vi "Day 2 - part a solution.vi"() -> ()   [LabVIEW 2020]
panel:
  in  "Input":string="A Y\nB X\nB X\nC Y\nB X\nA Z\nB X\nB X\nC Z\nA Z\nC Z\nA X\nA Y\nA Y\nB X\nC Y\nB Z\nA X\nB X\nC Y\nC Y\nA Y\nA Y\nC Y\nB X\nB X\nB X\nA X\nB X\nB X\nC Y\nC Y\nB X\nA Z\nA Z\nB X\nA Z\nC Y\nB X\nB X\nB X\nB X\nB X\nB Z\nA Z\nB X\nA Z\nA X\nB X\nA Z\nB X\nC Y\nA Z\nA Z\nB X\nB X\nB Z\nC Y\nA Y\nB Z\nA Z\nC Z\nB X\nC Y\nC Y\nB Z\nB X\nB X\nB Z\nB X\nB X\nA Y\nA Z\nB Z\nB X\nB Y\nB Z\nB X\nC X\nB Z\nB X\nA Z\nB Z\nB Z\nB X\nA Y\nA Z\nA Y\nB X\nB Z\nB X\nB X\nA Y\nA Y\nB X\nB X\nB X\nC X\nC Y\nB X\nB X\nB Z\nB X\nB X\nB X\nC Y\nB X\nC Y\nA Z\nB X\nB Z\nB X\nC Y\nC Y\nA Z\nA Y\nC Y\nB X\nB X\nB Z\nA Y\nB X\nB X\nB X\nA Y\nB Z\nB X\nA Y\nB Z\nC Y\nA X\nB X\nB X\nA Z\nC Y\nB X\nB Z\nA Y\nA Y\nC Y\nA Y\nC Y\nB X\nB Z\nB X\nC Y\nA Y\nB X\nC Z\nA Z\nC Y\nB X\nB Z\nB X\nB X\nB Z\nB Y\nA Y\nB X\nA Y\nA Z\nA Z\nB X\nC Y\nB Z\nA X\nA Y\nB X\nA Z\nB X\nA Y\nB Y\nB X\nA Y\nB X\nB X\nB X\nB X\nB X\nB X\nB X\nA Z\nB X\nB X\nB Z\nB Z\nB Z\nB Z\nA Y\nB Z\nC Z\nB X\nB X\nB X\nA Z\nB Z\nC Y\nB X\nC Y\nB Z\nB X\nB Z\nB X\nC Z\nA Z\nA Y\nA X\nB X\nB Z\nA Y\nB X\nB X\nB X\nB X\nC Y\nC Y\nA Z\nA Y\nA X\nB X\nB X\nA Y\nB X\nC Y\nA X\nB X\nB X\nB X\nA Z\nC Y\nB Z\nC Y\nA Y\nC Y\nA X\nA Z\nC Z\nA Z\nB X\nB Z\nB X\nB X\nA X\nB X\nB X\nB Z\nA Y\nC Y\nA Z\nC Z\nA Z\nA Z\nA Z\nB Z\nB Z\nB Z\nC Z\nB Y\nC Y\nC Y\nC X\nB X\nC Y\nB X\nB X\nC Y\nB Z\nB X\nC Z\nB X\nA Z\nB Z\nC X\nC Y\nB X\nA Y\nA Z\nB X\nA Z\nA Z\nB X\nB X\nC Z\nB Z\nA Z\nA Z\nC Z\nB X\nA Z\nA X\nB X\nB X\nC Y\nB X\nB Z\nA Z\nB X\nB X\nB X\nB X\nB X\nB X\nB X\nB X\nC Y\nC Y\nB X\nB X\nB X\nC Y\nA X\nB Z\nB X\nB X\nC Z\nB X\nB Z\nB Z\nA Z\nB X\nB Z\nB X\nA Z\nB X\nB X\nB X\nB X\nB X\nC Z\nB X\nB X\nB X\nB Z\nC Y\nC Y\nA Y\nB X\nB Z\nC Y\nB X\nB X\nC Y\nC Y\nB X\nB X\nB X\nB X\nC X\nB Z\nB X\nB Z\nC Y\nA X\nA Z\nB X\nB X\nA Z\nB X\nC Z\nB X\nA Y\nA Z\nB X\nB X\nB X\nB Z\nB X\nA Y\nC Y\nB Z\nB Z\nC Y\nB X\nA Y\nC Y\nB X\nC Z\nB X\nB X\nA Z\nB Z\nB Z\nB X\nA Z\nA Z\nA Y\nB Z\nB X\nB X\nB X\nB X\nB Z\nB X\nB Z\nB X\nA Z\nB X\nB X\nC Z\nC Z\nB X\nC Y\nA Z\nB X\nB Z\nC Z\nC X\nB X\nA Y\nA Y\nB X\nB X\nC Y\nA X\nC Y\nA Y\nA Z\nC Z\nB Z\nA Z\nB X\nB X\nB Z\nC Y\nA Y\nA Y\nB Z\nA Z\nA Z\nB Z\nA Z\nB X\nA Y\nA Y\nC Y\nB X\nB X\nA X\nB X\nC X\nA Y\nA Z\nB X\nB X\nB X\nB X\nB X\nB Z\nB Z\nB Z\nB X\nB X\nA Z\nB X\nC Z\nA Z\nC Y\nB Z\nC Y\nA Y\nC Y\nB X\nB X\nB X\nA Y\nB Z\nB Z\nB X\nB Z\nB X\nB X\nB X\nC Y\nB X\nB Z\nA Z\nB X\nB X\nB X\nC Z\nC Z\nB Z\nB X\nA Z\nA X\nB X\nB X\nB Y\nA Y\nB X\nB X\nC Z\nA Z\nB X\nB Z\nB Z\nA Y\nA Z\nB Z\nB Z\nA Y\nA Y\nA Z\nC Y\nC Y\nB X\nB X\nA Z\nB X\nC Y\nC X\nA Z\nB X\nB X\nB X\nA Y\nC Y\nB Y\nC Y\nC X\nA X\nA Y\nB Z\nB X\nB Z\nA X\nB X\nC Z\nB X\nB X\nA Y\nB Z\nB X\nA Y\nA Y\nB X\nC Y\nB X\nB X\nC Y\nB X\nC Z\nB Z\nB X\nA X\nC Y\nC Y\nB X\nB Z\nB X\nB X\nA Z\nB X\nA Z\nB Z\nB X\nB X\nB Z\nA Y\nC Y\nB Z\nB X\nA Y\nB X\nA X\nC Z\nB X\nB Z\nB Z\nA X\nC Y\nA Z\nB X\nB Z\nA Y\nB X\nC Y\nA Y\nB Z\nC Y\nB X\nB X\nB X\nB X\nB X\nB X\nC Y\nB X\nC Z\nA Y\nC Y\nB X\nC Y\nB Z\nB X\nA X\nB Z\nB X\nC X\nB X\nA Z\nB X\nA Y\nB X\nC Z\nB X\nB Z\nA Y\nB X\nA Z\nA Z\nA Z\nA Y\nA Y\nB X\nA Z\nB X\nB X\nA Y\nA Y\nA Y\nB Z\nC Y\nB Z\nB X\nC Z\nA Y\nC Y\nB X\nB X\nB Z\nB X\nB X\nB X\nC Y\nC Y\nA Y\nB Z\nB Z\nB X\nB X\nB Z\nB X\nA Y\nC Y\nB X\nC X\nB Z\nB X\nB Z\nB Z\nC Y\nB Z\nB X\nC X\nB X\nC Y\nB X\nA Z\nB X\nB X\nB X\nB X\nB X\nC Y\nA Y\nB X\nC Y\nB Z\nB Z\nB X\nC X\nB Z\nC Y\nC X\nC Y\nA Z\nB Z\nC Y\nC X\nB X\nA Y\nC Y\nB X\nC Z\nB Z\nA Y\nC Z\nC X\nB X\nB X\nA Y\nC X\nB X\nB X\nA X\nA Z\nA X\nA Y\nA Y\nC Y\nB X\nC Z\nB X\nC Y\nA Y\nB X\nB X\nB X\nB X\nA Z\nC X\nB X\nB Z\nB X\nB X\nC Y\nB X\nC Z\nB X\nB X\nB X\nB X\nB X\nC Y\nB X\nB X\nA Y\nB X\nC Y\nC Y\nA Y\nB X\nA X\nA Y\nB X\nB Z\nB X\nB Z\nA X\nA Y\nA X\nB X\nC Z\nA Y\nB Z\nA Y\nB Z\nB Z\nB X\nB Z\nB X\nB X\nB X\nB Z\nB X\nB X\nB X\nA Z\nC Z\nC Z\nA X\nA X\nB X\nB X\nA X\nB X\nA X\nA Z\nB Z\nB X\nC Y\nB X\nC Y\nA Y\nC X\nA X\nA Y\nB Z\nB X\nB X\nC Z\nB Y\nA Y\nB Y\nC Y\nA Y\nB X\nB X\nC X\nB Z\nA Y\nB Z\nA Z\nB X\nB X\nA Z\nC Z\nA Y\nB X\nB X\nB Z\nB X\nB X\nB Z\nA X\nA Z\nC Y\nA Y\nA Z\nB X\nC Y\nB Z\nC Y\nB X\nB X\nB Z\nB X\nA Y\nB X\nA Y\nB X\nA Y\nB X\nA Y\nC Y\nA Y\nB Z\nA Y\nB X\nA Z\nC Y\nB X\nB X\nB X\nA X\nB X\nB Z\nA Z\nA Z\nB X\nB Z\nB X\nA Y\nB Z\nB X\nB X\nA Y\nA Y\nC Z\nC Y\nB X\nA X\nA Y\nA X\nC Y\nB X\nC X\nB X\nB X\nA Y\nA Y\nA Y\nB Y\nB X\nB X\nB X\nC Z\nB Z\nC Z\nA X\nB X\nB X\nA Y\nA Z\nB X\nA Y\nB Z\nB Z\nC Y\nB X\nB X\nC X\nB X\nC X\nB X\nB Z\nA X\nB X\nA Z\nA X\nB Z\nA Y\nB X\nB X\nB X\nB X\nB Z\nA Z\nB X\nB Z\nB X\nB Z\nC Y\nB X\nC Y\nB X\nB X\nB X\nA Y\nB X\nA Y\nB X\nB X\nA X\nC Z\nC Y\nA Z\nB X\nA Y\nC Z\nC Y\nC Y\nB Z\nA Y\nB X\nA Y\nB X\nB X\nB Z\nB Z\nB X\nC X\nB Z\nA X\nA Y\nA Y\nB Z\nA Z\nC Y\nB X\nB Z\nA Y\nC Y\nA Y\nA X\nA Z\nB X\nB X\nC Y\nB X\nC Y\nB X\nA X\nB Z\nC X\nB Y\nA Y\nC Y\nB X\nA X\nB X\nB X\nB X\nA Z\nA Y\nB X\nC Z\nB X\nC X\nC Z\nB X\nB X\nC Y\nB X\nB Z\nA Y\nA Y\nB X\nB X\nB Z\nC Y\nB X\nB X\nB X\nA Y\nC Y\nB X\nA Y\nA Z\nC Y\nB X\nA Y\nA Z\nB Z\nA Z\nB X\nC X\nB Z\nA Y\nB Z\nA Y\nC Y\nA X\nA Y\nB X\nC Y\nC Y\nB X\nA X\nB Z\nB X\nB X\nA Z\nA Z\nA Y\nA Y\nB X\nB X\nB X\nA X\nB X\nB X\nB X\nA X\nB Z\nC Z\nA Y\nC Y\nC Y\nC X\nB X\nB Z\nB Z\nB X\nB X\nC Y\nA X\nC Y\nA X\nB X\nB X\nB Z\nB Z\nC Y\nC Y\nA Z\nC Y\nA Z\nB X\nA Z\nA Y\nB Z\nB Z\nB X\nB X\nA Y\nB Z\nB X\nC Z\nA Z\nB Z\nB X\nB Z\nB X\nC Y\nB X\nA Y\nB Z\nC Y\nB Z\nC Z\nB X\nC Z\nB X\nB X\nB X\nC Y\nB X\nB X\nB Z\nA Y\nB X\nB Z\nA Z\nB X\nC Y\nC X\nC Y\nA Z\nB X\nA Z\nB X\nC Z\nA Y\nB Z\nB Z\nA Y\nC Z\nC X\nA Y\nB X\nB Z\nB X\nB X\nB X\nB X\nA X\nB X\nB X\nA Z\nB X\nB X\nA Z\nC Y\nA X\nB Z\nB X\nB X\nA Z\nB X\nA Y\nB Z\nC Y\nB X\nA Y\nC Y\nB Z\nB X\nA Z\nA Z\nB X\nB X\nB Z\nB X\nB X\nA Z\nB X\nB Z\nB Z\nC Y\nA Z\nB X\nA Y\nB X\nB X\nB X\nB Z\nA X\nC Y\nB Z\nB X\nB X\nB X\nB X\nB X\nB Z\nB X\nB Z\nA Z\nB Z\nB X\nC Z\nB Z\nC Z\nA Z\nC X\nA Y\nB Z\nB Z\nB X\nB Z\nB Z\nA Z\nC Z\nA X\nC Y\nC Y\nA Y\nA X\nA Z\nB X\nA Y\nB X\nB X\nC Y\nC Y\nB X\nB Z\nA Y\nB X\nB Z\nB X\nB X\nA Z\nC Y\nB X\nC Y\nA Y\nB Z\nA Z\nA Y\nB X\nA Z\nB Z\nB X\nA Y\nA Y\nA Z\nA X\nB Z\nC Z\nB X\nC Z\nB X\nB Z\nA X\nB X\nB X\nB X\nB X\nC Y\nB X\nA X\nB Z\nA Y\nB X\nA Z\nB X\nB Z\nA Y\nA Y\nA Y\nA Y\nA Z\nC Y\nC Z\nB X\nB Z\nA Y\nB X\nB X\nB X\nA Y\nB Z\nB X\nB Z\nB X\nB X\nB X\nC Y\nC Y\nC X\nB X\nA Y\nA Y\nC Z\nA Y\nA Y\nC X\nA Z\nB X\nB X\nB X\nB X\nC Y\nA Y\nB Z\nA Z\nB X\nC X\nA Z\nB X\nC Y\nB X\nB X\nC Y\nB X\nB X\nB X\nA Y\nB X\nB X\nC Z\nB X\nC Y\nC Y\nB X\nA Z\nB X\nB X\nC Y\nA Y\nB X\nB Z\nB X\nB X\nB X\nC Y\nC Z\nB Z\nC Y\nB X\nB Z\nB X\nB X\nB X\nC Y\nC X\nB X\nA Y\nA Z\nB Z\nA Y\nB X\nB X\nB Y\nC Y\nC X\nB Z\nA Z\nB X\nB X\nA Y\nC Z\nC Y\nB X\nC Y\nA Z\nA Y\nB Z\nB X\nB X\nB X\nB X\nA Z\nA X\nA X\nA X\nC Y\nB Z\nB X\nC Y\nB X\nB X\nA Z\nC Z\nC Z\nB X\nA Y\nB X\nB Z\nB X\nA Y\nA Y\nA Z\nC Y\nA Y\nA Z\nA Y\nA Y\nB X\nA Y\nB X\nA Z\nA Z\nC Y\nB X\nB X\nC Y\nB X\nB X\nB X\nC Y\nA Y\nB X\nA Y\nB Z\nC Y\nB X\nA Y\nB Z\nA Z\nB Z\nA Z\nB X\nC Y\nB X\nB X\nB X\nC Y\nA Y\nB X\nA Y\nC X\nA Z\nB X\nB Y\nB X\nB X\nA Z\nB X\nB X\nB Z\nB X\nC Y\nB X\nB X\nB Z\nB X\nC Y\nB X\nC Y\nB X\nB Z\nA Y\nB X\nB X\nC Z\nB X\nC Y\nA Y\nC Y\nB X\nB Z\nB X\nB X\nB X\nB X\nA Y\nB X\nA Z\nA Y\nA X\nC Y\nB X\nC Y\nB X\nA Z\nC Y\nC Y\nB Z\nB X\nA Y\nB Z\nA Y\nA Y\nB Z\nB Z\nB X\nC Y\nC Y\nB X\nA X\nA Z\nB X\nC Y\nB X\nB X\nB Z\nB X\nB Z\nC Y\nC Z\nC Y\nA Y\nA Z\nB X\nC Y\nA Y\nC X\nB X\nB X\nA Y\nB X\nB X\nB X\nB Z\nB Y\nA X\nA Y\nC Y\nC Y\nA Y\nC Y\nB Z\nB Z\nC Y\nB X\nC Y\nC Z\nA Y\nC X\nA Y\nA Y\nC Y\nC Y\nB X\nA Y\nA X\nB X\nB X\nB Z\nB X\nA Z\nA Y\nA Y\nB X\nB X\nB Z\nB Z\nB X\nB Z\nA Z\nA Y\nA Z\nB X\nC Y\nB Z\nB X\nA Y\nB X\nC X\nB X\nB X\nC Y\nB X\nB X\nB X\nA Y\nA X\nA Y\nB X\nB X\nA Y\nA Y\nA Z\nA Z\nC X\nC Y\nA Z\nC Y\nB Z\nB X\nA Y\nB X\nB Z\nC Z\nA Y\nA Z\nA Y\nB X\nB Z\nB X\nA X\nB Z\nB X\nC Y\nB X\nA Z\nC Z\nA X\nB X\nB X\nA Y\nC Y\nB X\nB X\nB X\nB X\nB X\nA X\nB X\nA Z\nC Z\nB Z\nB X\nC X\nA X\nC Y\nA Y\nA Z\nB X\nA X\nA Z\nA Z\nB X\nB X\nA Z\nC Y\nA Z\nB X\nC Y\nB X\nC Z\nC Y\nC X\nA Z\nC X\nB Z\nB X\nB X\nC Y\nB X\nC Y\nA Z\nA Z\nA Z\nA Y\nA Z\nB X\nB X\nB X\nB Z\nC Y\nC Z\nC Y\nC Y\nC Y\nA Y\nB Z\nA X\nB X\nB X\nB X\nA X\nA Y\nB X\nB Z\nA Z\nA Y\nA Y\nB Z\nB X\nB X\nC Y\nC Y\nC Y\nB X\nC Y\nB X\nB X\nB X\nC Y\nA Y\nA Y\nC Z\nC Y\nB X\nA X\nA Y\nB X\nC Y\nB X\nA Y\nC Y\nA Y\nB X\nB X\nB Z\nA Y\nB Z\nB Z\nB X\nB X\nC X\nC Y\nB X\nB X\nA X\nC Y\nB X\nB Z\nB X\nB X\nA Y\nB X\nB Z\nB Z\nC Y\nB X\nB Z\nB Z\nB Z\nB X\nB X\nA Y\nB X\nB X\nB Z\nC Y\nA Y\nB X\nB Z\nB X\nB X\nA X\nB X\nB X\nB X\nB Z\nB Z\nB Z\nB X\nA Z\nB X\nA Z\nA Y\nB Z\nB X\nA Y\nB X\nB Z\nB X\nA Z\nB X\nB Z\nC Z\nA X\nB X\nB X\nB X\nC Y\nB X\nB X\nA Y\nA Z\nB X\nC Y\nB X\nC Y\nB X\nB Y\nB X\nC Z\nB X\nC Z\nA Y\nB X\nC Z\nB X\nA Y\nC Y\nB X\nB X\nB Z\nC X\nB Z\nB X\nA Z\nB X\nB X\nB X\nB Z\nB X\nA Z\nC Y\nA Y\nB X\nB X\nA Z\nB X\nA Y\nB X\nC Y\nB Z\nB Z\nB X\nB Z\nB X\nB X\nB X\nB X\nB X\nC Y\nA Z\nA Z\nB Z\nA Y\nB Z\nC Y\nA Y\nA Y\nC Y\nA Y\nB Z\nA Y\nA Y\nB X\nB X\nA X\nB X\nC Y\nC Y\nB Z\nB X\nA Z\nB Z\nB X\nA Z\nB Z\nA Y\nA Y\nA Y\nA Y\nA Z\nA Y\nB X\nB Z\nA Y\nB X\nA Z\nB Z\nC X\nB X\nB X\nB Z\nB Z\nB X\nB X\nB X\nB X\nB X\nB X\nB X\nB Z\nB X\nB X\nB X\nB X\nB X\nB Z\nB X\nB X\nB Z\nB Z\nB X\nA Y\nB Z\nB X\nA Z\nA Y\nA Z\nB X\nB X\nA X\nB Y\nA Z\nB X\nC Z\nA Z\nB X\nB Z\nB X\nB X\nB X\nA Y\nC Y\nB X\nB X\nB X\nA Y\nB X\nA Z\nB X\nB X\nB X\nB Z\nB Z\nC X\nC Y\nB X\nB X\nC Y\nB X\nB X\nB X\nA X\nA Z\nA Z\nB Z\nB Z\nB X\nA Y\nB X\nC Y\nB Z\nC Y\nC Z\nA Y\nA Y\nB X\nB X\nA Z\nB X\nB X\nB Z\nB X\nB X\nA Z\nB X\nB X\nB X\nC Y\nB X\nB X\nC Y\nB X\nB X\nB Z\nB X\nB X\nA Y\nC Y\nA X\nC Y\nB X\nB X\nA Z\nA Y\nB X\nA X\nB Z\nA Y\nB X\nB X\nA Y\nB X\nC X\nB X\nB X\nB Z\nB Z\nB X\nB Z\nB X\nB X\nA Y\nA Y\nB X\nB Z\nC Y\nB X\nB X\nB X\nA Z\nB X\nA Y\nB X\nC Y\nA X\nA Y\nB X\nB X\nC Y\nB X\nB X\nB X\nA Z\nB Z\nB X\nC X\nA Z\nC Y\nB X\nB Z\nB X\nB X\nA Z\nB X\nA Y\nC Y\nB X\nB Z\nC X\nA Z\nA Z\nB Z\nB Z\nA X\nB X\nA Y\nB X\nB X\nB X\nB X\nA Z\nB Z\nB Z\nC Y\nA X\nA Y\nA Y\nA Z\nB X\nA Y\nB Z\nC Y\nB Z\nB X\nA Z\nB Z\nB X\nB Z\nB Z\nB Z\nB X\nC Y\nB X\nB X\nA Y\nB X\nC X\nA Y\nA Z\nA Y\nB X\nC Y\nB Z\nB X\nB X\nA X\nB X\nB X\nA Y\nA Z\nC Z\nA Y\nB X\nB X\nC Y\nA X\nA Z\nB X\nB Z\nB Z\nC Y\nA Z\nC Y\nA Z\nC Y\nC Y\nB Z\nC Y\nB X\nC Y\nC Y\nB X\nB Z\nC X\nC Y\nA Y\nB X\nC Y\nB X\nB X\nC Y\nB Z\nB Z\nA Z\nA Z\nC Y\nB X\nB Z\nB X\nB X\nB X\nC Y\nB X\nC Y\nA Z\nA Z\nB X\nB X\nA Y\nA X\nB X\nA Z\nA Y\nC Y\nB X\nA Y\nA Y\nB X\nA X\nA Z\nA Y\nA Z\nC Y\nC Y\nC Y\nA Y\nB X\nB X\nA Y\nC Y\nB X\nA X\nC Y\nC Y\nA Y\nC Y\nC Y\nB Z\nC Y\nB X\nC Y\nB X\nB X\nB X\nA Y\nB Y\nB X\nC X\nB X\nA X\nA Y\nC Y\nC Y\nB X\nB X\nA Y\nB X\nB X\nA Y\nC Y\nC X\nA Y\nB X\nB Z\nB Z\nB Z\nB X\nA Z\nB X\nB X\nA Y\nB X\nB X\nA Y\nB Z\nA Y\nB X\nB X\nB Z\nA Z\nA Y\nA Z\nA Y\nC Y\nB X\nC X\nB X\nB X\nA Z\nB X\nB Z\nB X\nA Z\nC Y\nB X\nB X\nB Z\nA Z\nA Y\nB X\nB Y\nA Y\nA Z\nA Y\nC Z\nB X\nB X\nB X\nA Z\nB X\nB X\nB X\nA Y\nB Z\nC Y\nC Y\nA Z\nA Z\nA Y\nB X\nA Y\nB Z\nC Y\nB X\nB Z\nA Y\nB X\nA Y\nC Y\nB X\nB X\nA Y\nA Z\nA Z\nA Z\nB X\nB X\nA Z\nB X\nB X\nB Z\nA X\nB Z\nA Z\nB X\nC Y\nC X\nA Z\nB X\nA Y\nB Y\nB Z\nB X\nB X\nA Y\nB X\nA Z\nA Z\nC X\nB X\nB Z\nA Y\nC Y\nA Y\nB X\nB Z\nB X\nA Z\nB Z\nC Y\nB Z\nB X\nB X\nB X\nA Y\nB X\nB X\nA Z\nC Y\nB X\nC Y\nB X\nC Y\nA Z\nA Y\nA X\nC Y\nB X\nB X\nB Z\nB X\nA Y\nA Y\nB X\nB X\nA Z\nC Y\nB Z\nB X\nB X\nA X\nA Y\nB Z\nC Y\nA Z\nC Y\nA Z\nB X\nA Y\nB X\nA Y\nB X\nB X\nC X\nB Y\nC Z\nA Z\nC Y\nB X\nB X\nB Z\nC Z\nA X\nA Y\nA Z\nB X\nC Y\nB Z\nB Z\nA Y\nB X\nB X\nA Y\nA Z\nB X\nB X\nA Z\nB X\nB X\nB Z\nA X\nB X\nA X\nA Y\nC Y\nB X\nB Z\nA Y\nB X\nA X\nB X\nB X\nB Z\nB X\nB X\nA Y\nB X\nB X\nA Y\nA Y\nC Y\nB Z\nB X\nA X\nA Z\nB X\nB X\nC Z\nB X\nB X\nB X\nB X\nB X\nC Y\nC Y\nC X\nB X\nB X\nB Z\nB Z\nB X\nA Y\nB Z\nB Z\nB Z\nB X\nB X\nB X\nB X\nA Y\nA Y\nB X\nC Y\nC Y\nB X\nB X\nA Y\nC Y\nA Z\nC Y\nB X\nC Z\nB X\nB Z\nB X\nC Y\nC Y\nB X\nB X\nB X\nC Y\nB X\nB X\nA X\nB X\nC Y\nA Y\nB X\nB X\nB X\nC X\nC Y\nA Y\nB X\nB X\nC Y\nA Y\nB X\nA Y\nA Y\nB Z\nC Y\nB Z\nA Y\nA Z\nC Y\nB X\nC Y\nB X\nC Y\nC Y\nB X\nB X\nB X\nB Z\nA Y\nB X\nB X\nB X\nA Y\nB X\nB X\nA Y\nB X\nA Y\nC Y\nA Z\nB X\nB X\nC Y\nB X\nB X\nA Y\nA Z\nC Y\nB X\nB Z\nB Z\nB X\nC Y\nB X\nA Y\nC X\nC Y\nB X\nB X\nB Z\nC Y\nB X\nB X\nC Y\nC Y\nB X\nC Y\nB Z\nC Y\nC X\nB Z\nC Y\nB Z\nC Y\nA X\nB Z\nB Z\nB X\nB X\nC Y\nB X\nC Y\nB X\nB X\nB X\nA Y\nB X\nC Y\nB Z\nC Y\nC Y\nA Y\nC Z\nA Y\nB X\nA Z\nC Z\nC Y\nB X\nB X\nA Y\nB Z\nB X\nC Y\nB X\nB Z\nA Z\nB Z\nA Y\nC Y\nA Z\nB X\nB X\nC Y\nC Y\nB X\nB X"
  out "sum":i32
  # "Advent of code day 2 pt A"
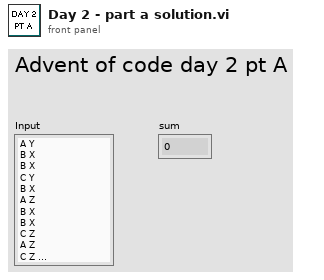
[diagram p1: front panel]
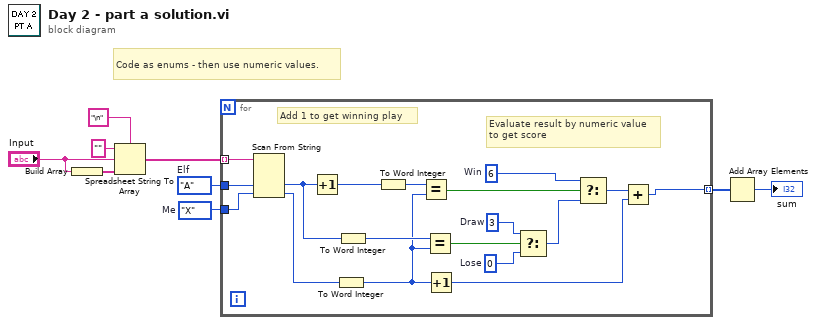
[diagram p0: block diagram]
diagram:
  w2 = enum16{"X", "Y", "Z"}."X"  # Me
  w1 = enum16{"A", "B", "C"}."A"  # Elf
  # "Code as enums - then use numeric values."
  n1 = Build Array("Input") -> (w9:string[])
  n2 = Spreadsheet String To Array(delimiter (Tab)="\n", format string="", spreadsheet string="Input", array type (2D Dbl)=w9) -> (array=w6:string[])
  n3 = for {
    tunnel: w6 -> [w27] mode=indexing
    tunnel: [w15] -> w4 mode=indexing
    tunnel: w2 -> [w11]
    tunnel: w1 -> [w10]
    w18 = 0  # Lose
    w20 = 3  # Draw
    w23 = 6  # Win
    # "Evaluate result by numeric value\nto get score"
    # "Add 1 to get winning play"
    n4 = Scan From String(input string=w27, default 1=w10, default 2=w11) -> (output 1=w12:enum16{"A", "B", "C"}, output 2=w13:enum16{"X", "Y", "Z"})  [unwired: 3 in, 3 out]
    n5 = Increment(x=w12) -> (x+1=w26:enum16{"A", "B", "C"})
    n6 = To Word Integer(number=w13) -> (16bit integer=w16:i16)
    n7 = To Word Integer(number=w12) -> (16bit integer=w22:i16)
    n8 = To Word Integer(number=w26) -> (16bit integer=w25:i16)
    n9 = Equal?(x=w25, y=w16) -> (x = y?=w24:bool)
    n10 = Equal?(x=w22, y=w16) -> (x = y?=w21:bool)
    n11 = Increment(x=w16) -> (x+1=w14:i16)
    n12 = Select(t=w20, s=w21, f=w18) -> (s? t:f=w19:i32)
    n13 = Select(t=w23, s=w24, f=w19) -> (s? t:f=w17:i32)
    n14 = Add(x=w17, y=w14) -> (x+y=w15:i32)
  }
  n15 = Add Array Elements(numeric array=w4) -> (sum=→"sum":i32)
